vi "新清晰度MTF.vi"(0 "Image Pixels":u16[][](array[numeric]), 2 "path in":path, 5 "焦距选择":i32) -> (9 "水平Bre":dbl, 10 "垂直线对V":dbl, 11 "垂直Bre":dbl, 14 "水平线对V":dbl, 15 "Min value":dbl, 17 "X 坐标":dbl, 18 "Max value":dbl, 19 "Y坐标":dbl)   [LabVIEW 2016]
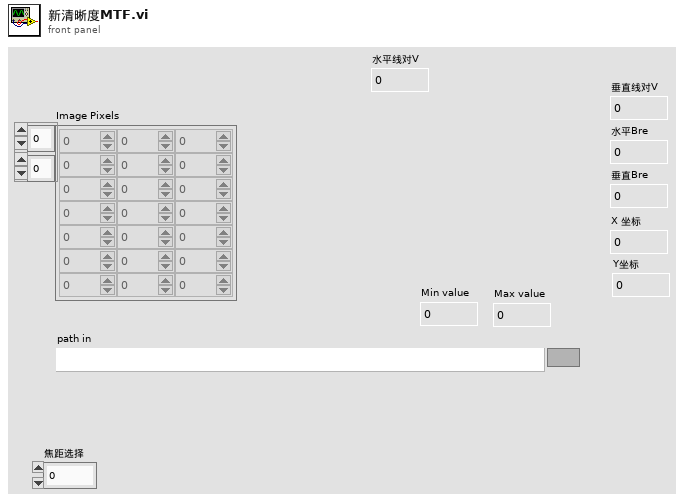
[diagram p1: front panel]
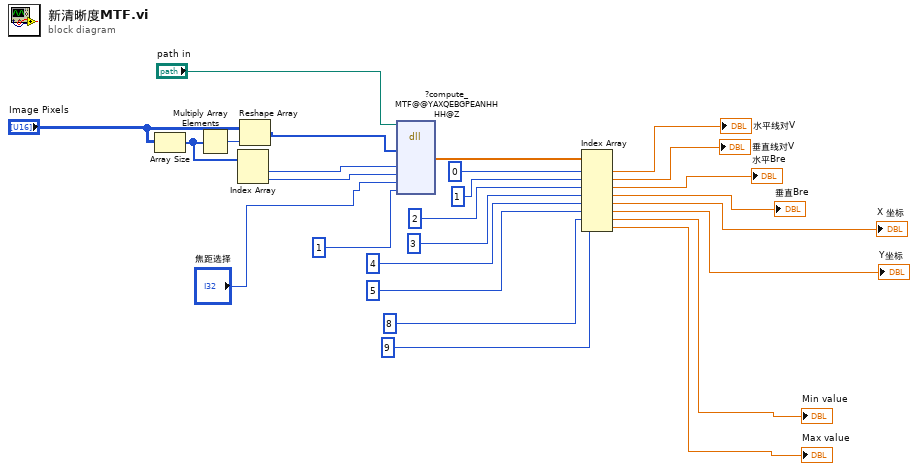
[diagram p0: block diagram]
diagram:
  n1 = Array Size(array="Image Pixels") -> (size(s)=w25:i32[])
  n2 = Multiply Array Elements(1:w25) -> (0:w23:i32)
  n3 = Index Array(array=w25) -> (element #1=w24:i32, element #2=w26:i32)  [unwired: 2 in]
  n4 = Reshape Array("Image Pixels", w23) -> (w16:u16[])
  n5 = dll-call lib="PTH2,abs HTiny1C出厂检测1dataxmtf.dll" fn="?compute_MTF@@YAXQEBGPEANHHHH@Z"(path in="path in", "im"=w16, "rows"=w24, "cols"=w26, "edge_strength_thr"="焦距选择", "number"=1) -> ("r"=w21:dbl[])  [unwired: 9 in, 2 out]
  n6 = Index Array(array=w21, index #1=0 ("index"), index #2=1 ("index"), index #3=2 ("index"), index #4=3 ("index"), index #5=4 ("index"), index #6=5 ("index"), index #7=8 ("index"), index #8=9 ("index")) -> (element #1=→"水平线对V":dbl, element #2=→"垂直线对V":dbl, element #3=→"水平Bre":dbl, element #4=→"垂直Bre":dbl, element #5=→"X 坐标":dbl, element #6=→"Y坐标":dbl, element #7=→"Min value":dbl, element #8=→"Max value":dbl)
